vi "zc_cz.vi"(0 "action":string, 1 "LabVIEW Web Service Request":refnum<class "Web Request.lvclass"> caption="LabVIEW Web服务请求", 2 "syren":string, 3 "sp_yijian":string, 4 "key":string, 5 "id":string, 7 "zc_luodi_num":string, 8 "sp_shuoming":string, 11 "fangshi":string, 12 "feiyong":string, 13 "shuoming":string, 14 "lc_num":string) -> (15 "error":errorcluster)   [LabVIEW 2017]
uses:
  <vilib>/wsapi/Web Request.lvclass
panel:
  in  "error 4":errorcluster={"status"=TRUE, "code"=254, "source"="您无权申请该流程！"} caption="error"
  in  "error 3":errorcluster={"status"=TRUE, "code"=255, "source"="当前资产不是“退出”状态！"} caption="error"
  out "postdata":string caption="post数据"
  out "error out":errorcluster caption="错误输出"
  # "Web服务请求输入接线端用于调用“Web服务”选板的VI。除非不需要访问该选板，否则不要在连线板上删除这个输入接线端。"
  # "添加至连线板的每一个其他输入控件，在URL中对应于一个输入。如需在接线端模式输出（默认设置）下包含显示控件，则该显示控件必须与连线板相连。"
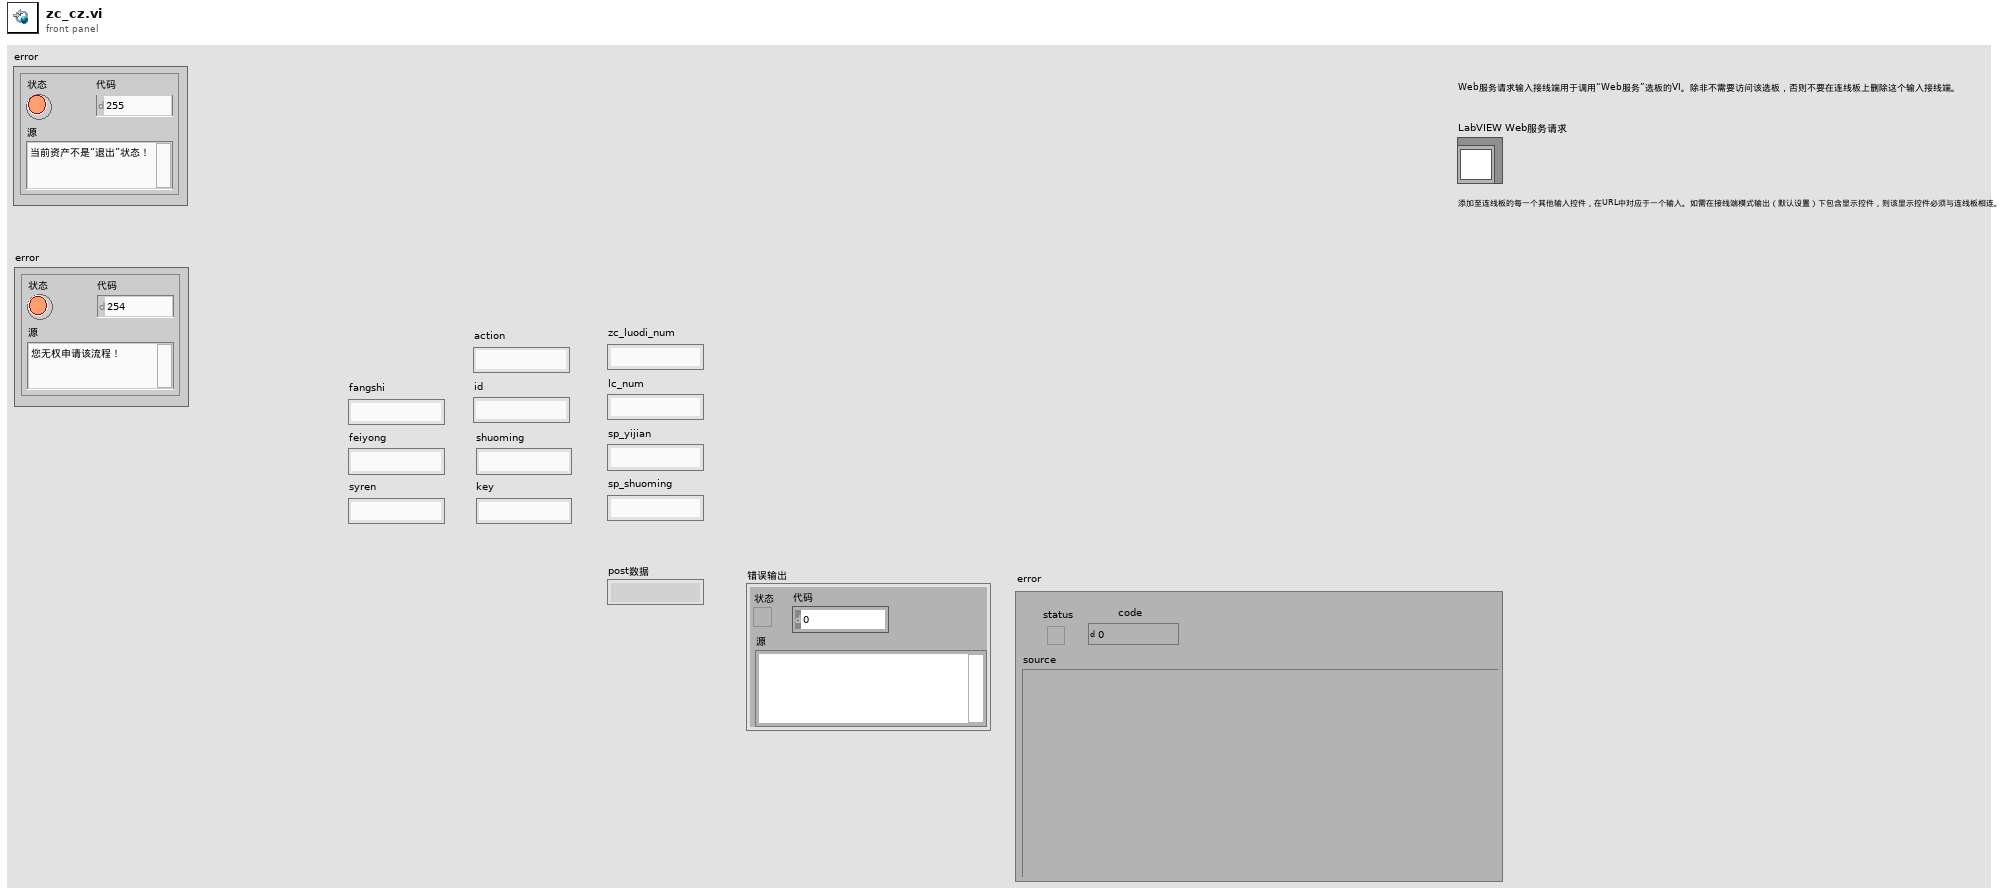
[diagram p1: front panel]
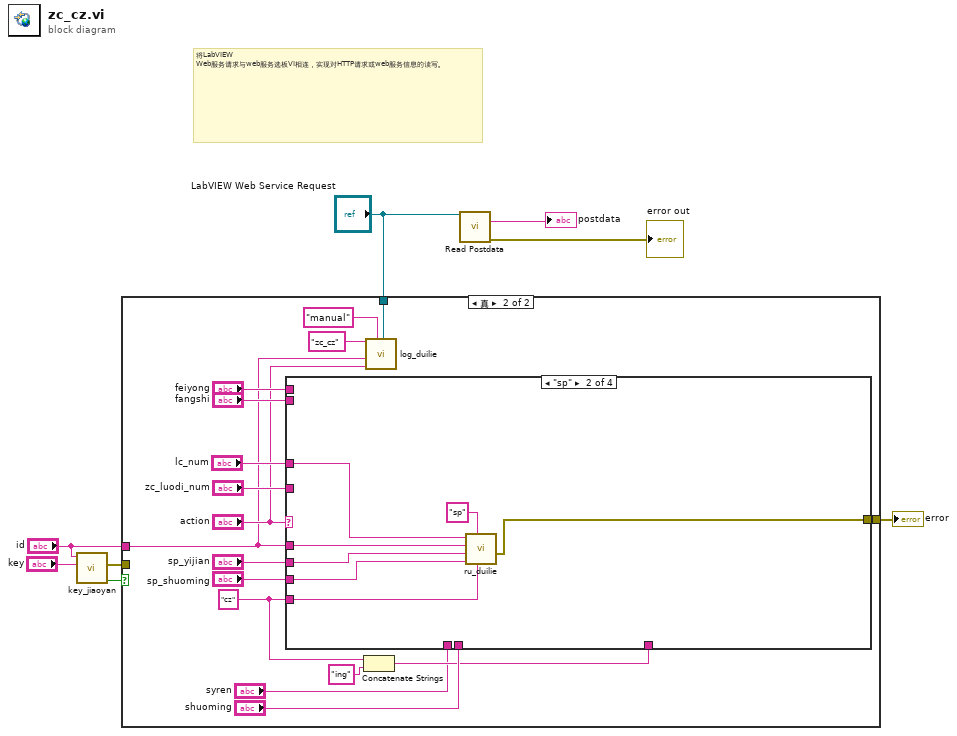
[diagram p0: block diagram]
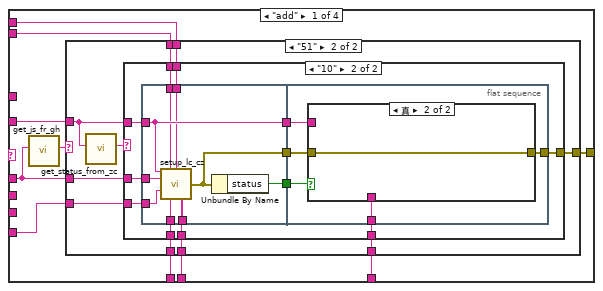
[diagram p3: hidden frame]
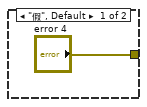
[diagram p4: hidden frame]
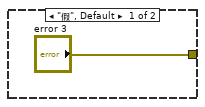
[diagram p5: hidden frame]
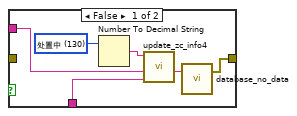
[diagram p6: hidden frame]
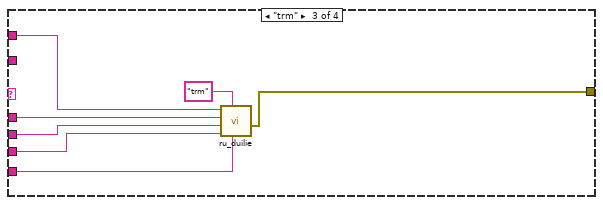
[diagram p7: hidden frame]
diagram:
  # "将LabVIEW Web服务请求与web服务选板VI相连，实现对HTTP请求或web服务信息的读写。"
  n1 = call "key_jiaoyan.vi"("key_client"="key", "gonghao"="id") -> ("jy"=w2:bool, "error"=w1:errorcluster)  [unwired: 8 in]
  n2 = case shown="真" w2 {
    tunnel: [w9 w21] -> w7
    tunnel: "LabVIEW Web Service Request" -> [_ w12]
    tunnel: "id" -> [_ w10]
    tunnel: w1 -> [w9 _]
    frame False {
    }
    frame True {
      w19 = "cz" ("yw")
      n3 = Concatenate Strings(w19, "ing" ("字符串")) -> (w18:string)
      n4 = case shown="\"sp\"" "action" {
        tunnel: w10 -> [w28 w87 w94 _]
        tunnel: "zc_luodi_num" -> [w29 _ _ _]
        tunnel: "sp_yijian" -> [_ w85 w92 _]
        tunnel: "sp_shuoming" -> [_ w84 w91 _]
        tunnel: "shuoming" -> [w36 _ _ _]
        tunnel: w19 -> [w35 w83 w90 _]
        tunnel: "lc_num" -> [_ w86 w93 _]
        tunnel: [w34 w82 w89 _] -> w21
        tunnel: w18 -> [w33 _ _ _]
        tunnel: "fangshi" -> [w32 _ _ _]
        tunnel: "feiyong" -> [w31 _ _ _]
        tunnel: "syren" -> [w30 _ _ _]
        frame "add" {
          n5 = call "get_js_fr_gh.vi"("gonghao"=w28) -> ("juese"=w27:string)  [unwired: 9 in, 1 out]
          n6 = case shown="\"51\"" w27 {
            tunnel: w36 -> [_ w47]
            tunnel: w35 -> [_ w46]
            tunnel: ["error 4" w45] -> w34
            tunnel: w33 -> [_ w44]
            tunnel: w32 -> [_ w43]
            tunnel: w31 -> [_ w42]
            tunnel: w30 -> [_ w41]
            tunnel: w29 -> [_ w40]
            tunnel: w28 -> [_ w38]
            frame "假", Default {
            }
            frame "51" {
              n7 = call "get_status_from_zc.vi"("zc_luodi_num"=w40) -> ("status"=w39:string)  [unwired: 9 in, 1 out]
              n8 = case shown="\"10\"" w39 {
                tunnel: w47 -> [_ w59]
                tunnel: w38 -> [_ w58]
                tunnel: w46 -> [_ w57]
                tunnel: ["error 3" w56] -> w45
                tunnel: w44 -> [_ w55]
                tunnel: w43 -> [_ w54]
                tunnel: w42 -> [_ w53]
                tunnel: w41 -> [_ w52]
                tunnel: w40 -> [_ w51]
                frame "假", Default {
                }
                frame "10" {
                  n9 = flat-sequence {
                    tunnel: w59 -> [w68]
                    tunnel: w51 -> [w65]
                    tunnel: w58 -> [w66]
                    tunnel: w57 -> [w67]
                    tunnel: [w65] -> w60
                    tunnel: w54 -> [w64]
                    tunnel: w53 -> [w63]
                    tunnel: w52 -> [w69]
                    tunnel: [w62] -> w50
                    tunnel: [w61] -> w49
                    tunnel: w60 -> [w72]
                    tunnel: [w74] -> w56
                    tunnel: w55 -> [w73]
                    tunnel: w50 -> [w71]
                    tunnel: w49 -> [w70]
                    frame #0 {
                      n10 = call "setup_lc_cz.vi"("zc_luodi_num"=w65, "fangshi"=w64, "feiyong"=w63, "id"=w66, "yw"=w67, "syren"=w69, "shuoming"=w68) -> ("error"=w61:errorcluster)  [unwired: 8 in]
                      n11 = Unbundle By Name(w61) -> ("status"=w62:bool)
                    }
                    frame #1 {
                      n12 = case shown="真" w71 {
                        tunnel: [w78 w81] -> w74
                        tunnel: w73 -> [w77 _]
                        tunnel: w72 -> [w75 _]
                        tunnel: w70 -> [_ w81]
                        frame False {
                          w76 = u8 130 items=["待验收"=1, "无需验收"=2, "验收不合格"=3, "待入库"=4, "入库"=5, "领用"=6, "借用"=7, "托管"=8, "接管"=9, "退出"=10, "出库在用"=11, "盘亏"=12, "出售"=13, "报废"=14, "领用中"=120, "退库中"=121, "借用中"=122, "归还中"=123, "转移中"=124, "调拨中"=125, "借调中"=126, "托管中"=127, "终止托管中"=128, "退出中"=129, "处置中"=130] ("状态选择器")
                          n13 = Number To Decimal String(number=w76) -> (decimal integer string=w79:string)  [unwired: 1 in]
                          n14 = call "update_zc_info4.vi"("ywxinxi"=w77, "number"=w75, "status"=w79) -> ("data_str"=w80:string)  [unwired: 8 in]
                          n15 = call "database_no_data.vi"("input"=w80) -> ("error"=w78:errorcluster)  [unwired: 2 in]
                        }
                        frame True {
                        }
                      }
                    }
                  }
                }
              }
            }
          }
        }
        frame "sp" {
          n16 = call "ru_duilie.vi"("yw"=w83, "name"="sp" ("元素"), "sp_shuoming"=w84, "sp_yijian"=w85, "id"=w87, "lc_num"=w86) -> ("error"=w82:errorcluster)  [unwired: 5 in]
        }
        frame "trm" {
          n17 = call "ru_duilie.vi"("yw"=w90, "name"="trm" ("元素"), "sp_shuoming"=w91, "sp_yijian"=w92, "id"=w94, "lc_num"=w93) -> ("error"=w89:errorcluster)  [unwired: 5 in]
        }
        frame Default {
        }
      }
      n18 = call "log_duilie.vi"("LabVIEW Web Service Request"=w12, "type"="manual", "action"="action", "user"=w10, "yw"="zc_cz") -> ()  [unwired: 7 in]
    }
  }
  "error" <- w7
  n19 = call <vilib>:"Read Postdata.vi"("LabVIEW Web Service Request"="LabVIEW Web Service Request") -> ("postdata"=→"postdata":string, "error out"=→"error out":errorcluster)  [unwired: 12 in, 1 out]
